vi "Calculate Saturator Dewpoint.vi"(8 "error in":errorcluster, 9 "RH_sat_out":dbl caption="RHsat (%)", 10 "Tair":dbl caption="Tair (degC)", 11 "RH_tar":dbl caption="RHtar (%)") -> (0 "error out":errorcluster, 3 "Td":dbl caption="Td (degC)" format="%.2f")   [LabVIEW 2014, in "Atmospheric Library.lvlib"]
doc: "This VI calculates the dewpoint at the outlet of a saturator which may be used as a water vapor source based on 1) the saturator outlet relative humidity <B>RH_sat_out</B>, 2) the temperature of air at the measurement point of interest <B>Tair</B> and 3) a desired RH at the measurement point of interest <B>RH_tar</B>. The value of saturator outlet humidity can account for non-ideal situations (in which the humidity at the saturator outlet is less than 100%), errors in temperature measurements and any losses in the system assuming that these values are constant with time. \n\nThe vapor pressures are calculated according to Murphy and Koop [2005]. Currently, the accessible range is 273 to 350 degC."
uses:
  Atmospheric Library.lvlib
  <vilib>/gmath/zero.llb/Ridders Zero Finder (VI).vi
  <vilib>/gmath/NI_Gmath.lvlib
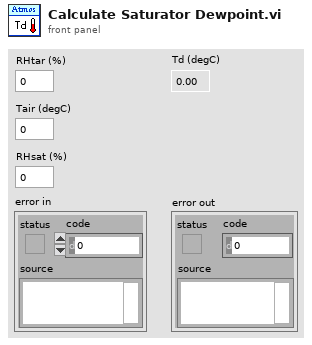
[diagram p1: front panel]
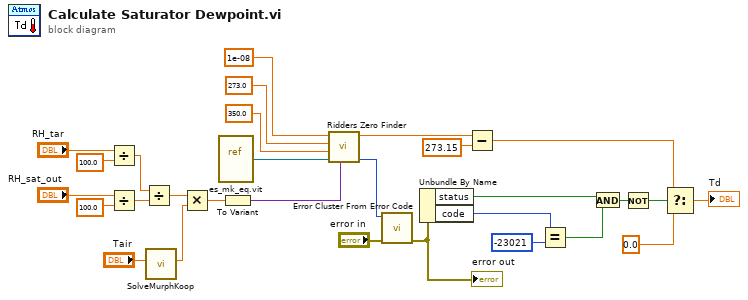
[diagram p0: block diagram]
diagram:
  n1 = Divide(x="RH_tar", y=100.0) -> (x/y=w25:dbl)
  n2 = Divide(x="RH_sat_out", y=100.0) -> (x/y=w24:dbl)
  n3 = Divide(x=w25, y=w24) -> (x/y=w23:dbl)
  n4 = call "SolveMurphKoop.vi"("T"="Tair") -> ("es"=w14:dbl)  [unwired: 7 in, 3 out]
  n5 = Multiply(x=w23, y=w14) -> (x*y=w21:dbl)
  n6 = vi-ref "es_mk_eq.vit"() -> (w22:refnum<vi>)
  n7 = To Variant(anything=w21) -> (Variant=w20:variant)
  n8 = call-poly <vilib>:"Ridders Zero Finder.vi"("data"=w20, "f(x)"=w22, "end"=350.0, "start"=273.0, "accuracy"=1e-08) -> ("error"=w12:i32, "zero"=w16:dbl)  [unwired: 3 in, 2 out]
  n9 = call <vilib>:"Error Cluster From Error Code.vi"("error in (no error)"="error in", "error code (0)"=w12) -> ("error out"=w10:errorcluster)  [unwired: 7 in]
  "error out" <- w10
  n10 = Unbundle By Name(w10) -> ("status"=w7:bool, "code"=w8:i32)
  n11 = Subtract(x=w16, y=273.15) -> (x-y=w3:dbl)
  n12 = Equal?(x=w8, y=-23021 ("code")) -> (x = y?=w6:bool)
  n13 = And(x=w7, y=w6) -> (x .and. y?=w5:bool)
  n14 = Not(x=w5) -> (.not. x?=w4:bool)
  n15 = Select(t=w3, s=w4, f=0.0) -> (s? t:f=→"Td":dbl)
